vi "Generate Ball Position.vi"() -> (3 "Array":T1(array[cluster]))   [LabVIEW 2025]
uses:
  <vilib>/Analysis/coordinate.llb/2D Cartesian Coordinate Rotation (Scalar).vi
  Framework/Robot Global Data.vi
  <vilib>/Analysis/NI_AALPro.lvlib
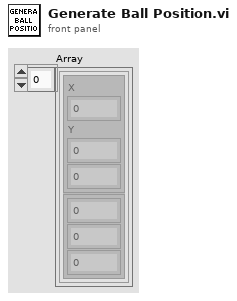
[diagram p1: front panel]
types:
  T1 = cluster{cluster{"X":dbl, "Y":dbl, dbl}, cluster{dbl, dbl, dbl}}[]
  T2 = cluster{"Ball Direction":dbl, "Ball Distance":dbl}[]
  T3 = cluster{cluster{"X":dbl, "Y":dbl, dbl}, cluster{dbl, dbl, dbl}}
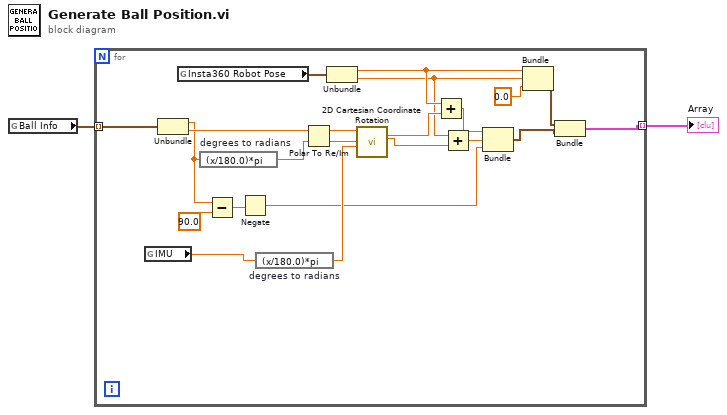
[diagram p0: block diagram]
diagram:
  n1 = global read "Robot Global Data.vi" "Ball Info"() -> (w2:T2)
  n2 = for {
    tunnel: [w5] -> w1 mode=indexing
    tunnel: w2 -> [w17] mode=indexing
    n3 = global read "Robot Global Data.vi" "IMU"() -> (w16:dbl)
    n4 = Unbundle(w17) -> ("Ball Direction"=w3:dbl, "Ball Distance"=w23:dbl)
    n5 = global read "Robot Global Data.vi" "Insta360 Robot Pose"() -> (w15:cluster{"X":dbl, "Y":dbl})
    n6 = expression code="(x/180.0)*pi" "degrees to radians"(w3) -> (w24:dbl)
    n7 = Subtract(x=w3, y=90.0) -> (x-y=w21:dbl)
    n8 = Negate(x=w21) -> (-x=w4:dbl)
    n9 = expression code="(x/180.0)*pi" "degrees to radians"(w16) -> (w18:dbl)
    n10 = Polar To Re/Im(2:w24, 3:w23) -> (0:w19:dbl, 1:w20:dbl)
    n11 = Unbundle(w15) -> ("X"=w11:dbl, "Y"=w9:dbl)
    n12 = call-poly <vilib>:"2D Cartesian Coordinate Rotation.vi"("theta"=w18, "y"=w19, "x"=w20) -> ("y out"=w10:dbl, "x out"=w12:dbl)  [unwired: 6 in, 1 out]
    n13 = Add(x=w11, y=w12) -> (x+y=w13:dbl)
    n14 = Add(x=w9, y=w10) -> (x+y=w8:dbl)
    n15 = Bundle(w13, w8, w4) -> (w6:cluster{dbl, dbl, dbl})  [unwired: 1 in]
    n16 = Bundle("X"=w11, "Y"=w9, 0.0) -> (w7:cluster{"X":dbl, "Y":dbl, dbl})  [unwired: 1 in]
    n17 = Bundle(w7, w6) -> (w5:T3)  [unwired: 1 in]
  }
  "Array" <- w1
